vi "日期字符串至簇.vi"(11 "字符串":string="2016-11-18") -> (0 "月内周":i32, 1 "日":i32, 2 "月":i32, 3 "年":i32)   [LabVIEW 2013, in "数据库操作.lvclass"]
panel:
  out "日":string
  out "月":string
  out "年":string
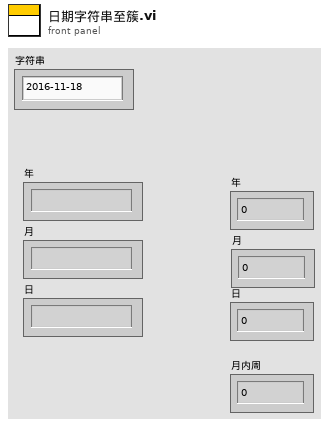
[diagram p1: front panel]
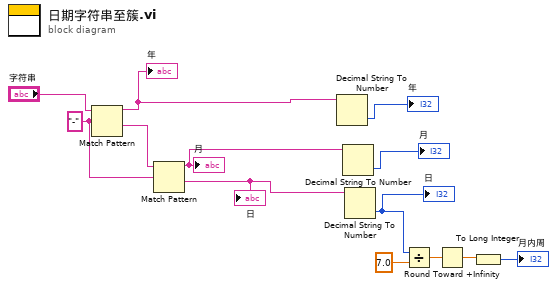
[diagram p0: block diagram]
diagram:
  w11 = "-" ("正则表达式")
  n1 = Match Pattern(string="字符串", regular expression=w11) -> (before substring=w10:string, after substring=w12:string)  [unwired: 1 in, 2 out]
  "年" <- w10
  n2 = Match Pattern(string=w12, regular expression=w11) -> (before substring=w9:string, after substring=w8:string)  [unwired: 1 in, 2 out]
  "月" <- w9
  "日" <- w8
  n3 = Decimal String To Number(string=w10) -> (number=→"年":i32)  [unwired: 2 in, 1 out]
  n4 = Decimal String To Number(string=w9) -> (number=→"月":i32)  [unwired: 2 in, 1 out]
  n5 = Decimal String To Number(string=w8) -> (number=w5:i32)  [unwired: 2 in, 1 out]
  "日" <- w5
  n6 = Divide(x=w5, y=7.0) -> (x/y=w3:dbl)
  n7 = Round Toward +Infinity(x=w3) -> (ceil(x): smallest int >= x=w2:dbl)
  n8 = To Long Integer(number=w2) -> (32bit integer=→"月内周":i32)
